vi "CAN Main.vi"(8 "error in (no error)":errorcluster, 10 "Interface":refnum<k21>="CAN1", 11 "Sequence Context In":refnum<k7>) -> (0 "error out":errorcluster)   [LabVIEW 2019, in "Wrappers.lvlib"]
uses:
  Wrappers.lvlib
  CAN/CAN.lvclass
  CAN/Setting.ctl
  <vilib>/addons/TestStand/_TSUtility.llb/TestStand - Set Property Value (Numeric Array).vi
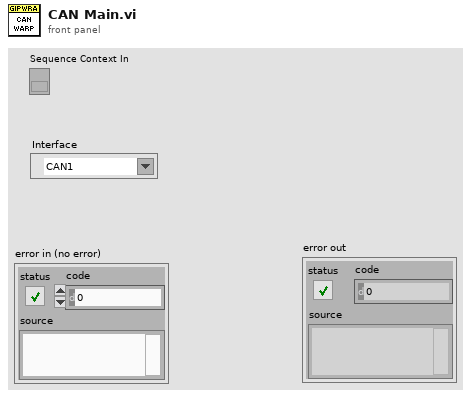
[diagram p1: front panel]
types:
  T1 = typedef "CAN.lvclass/Setting.ctl" = cluster{"Termination":u32, "Baud Rate":u64, "Interface":refnum<k21>, "XNET Database":refnum<k21>, "ECU":refnum<k21>}
  T2 = typedef "TestStand - Status Monitor.ctl" = cluster{"Sequence Context":refnum<k7>, "Execution":refnum<k7>, "Termination Monitor":refnum<k7>}
  T3 = cluster{"Send Tx":bool, "Stop":bool, "Rx Signals":string[], "Tx Signals":string[], "Tx Values In":dbl[]}
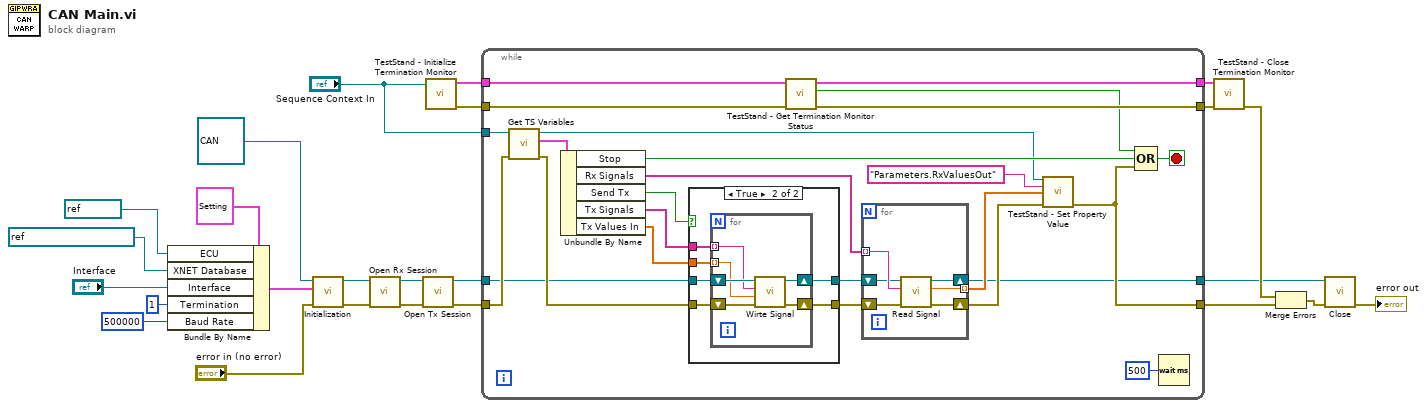
[diagram p0: block diagram]
diagram:
  n1 = Bundle By Name(cluster=T1 {"Termination"=1, "Baud Rate"=125000, "Interface"="CAN1", "XNET Database"="GIP_CAN_Database", "ECU"="GIP\nGIP_CAN_Database"} ("Setting"), "ECU"=refnum<k21> "GIP\ncan_messages_818", "XNET Database"=refnum<k21> "can_messages_818", "Interface"="Interface", "Termination"=u32 1, "Baud Rate"=u64 500000) -> (w11:T1)
  n2 = call "Initialization.vi"("error in (no error)"="error in (no error)", "Setting"=w11, "CAN in"=refnum<class "CAN.lvclass"> refnum ("CAN.lvclass")) -> ("error out"=w9:errorcluster, "CAN out"=w7:refnum<class "CAN.lvclass">)  [unwired: 7 in]
  n3 = call "Open Rx Session.vi"("error in (no error)"=w9, "CAN in"=w7) -> ("error out"=w8:errorcluster, "CAN out"=w6:refnum<class "CAN.lvclass">)  [unwired: 8 in]
  n4 = call "Open Tx Session.vi"("error in (no error)"=w8, "CAN in"=w6) -> ("error out"=w5:errorcluster, "CAN out"=w4:refnum<class "CAN.lvclass">)  [unwired: 8 in]
  n5 = call <vilib>:"TestStand - Initialize Termination Monitor.vi"("Sequence Context In"="Sequence Context In") -> ("error out"=w20:errorcluster, "Status Monitor Out"=w19:T2)  [unwired: 9 in]
  n6 = while {
    tunnel: w5 -> [w30]
    tunnel: w20 -> [w50]
    tunnel: w19 -> [w49]
    tunnel: [w48] -> w15
    tunnel: [w47] -> w18
    tunnel: "Sequence Context In" -> [w34]
    tunnel: [w42] -> w16
    tunnel: w4 -> [w29]
    tunnel: [w26] -> w1
    stop <- w46 stop-if-true
    n7 = call "Get TS Variables.vi"("error in (no error)"=w30, "Sequence Context In"=w34) -> ("error out"=w31:errorcluster, "Variables"=w32:T3, "Sequence Context Out"=w33:refnum<k7>)  [unwired: 7 in]
    n8 = Unbundle By Name(w32) -> ("Stop"=w43:bool, "Rx Signals"=w36:string[], "Send Tx"=w39:bool, "Tx Signals"=w40:string[], "Tx Values In"=w28:dbl[])
    n9 = case shown="True" w39 {
      tunnel: w31 -> [w52 w58]
      tunnel: [w52 w56] -> w38
      tunnel: w40 -> [_ w57]
      tunnel: w29 -> [w51 w55]
      tunnel: w28 -> [_ w54]
      tunnel: [w51 w53] -> w27
      frame False {
      }
      frame True {
        n10 = for {
          shift-right: [w63] -> w56
          shift-left: w58 -> [w64]
          tunnel: w57 -> [w61] mode=indexing
          tunnel: w54 -> [w60] mode=indexing
          shift-right: [w59] -> w53
          shift-left: w55 -> [w62]
          n11 = call "Wirte Signal.vi"("error in (no error)"=w64, "Signal Write"=w60, "Tx Signal In"=w61, "CAN in"=w62) -> ("error out"=w63:errorcluster, "CAN out"=w59:refnum<class "CAN.lvclass">)  [unwired: 6 in]
        }
      }
    }
    n12 = call <vilib>:"TestStand - Get Termination Monitor Status.vi"("error in (no error)"=w50, "Status Monitor In"=w49) -> ("error out"=w48:errorcluster, "Terminating or Aborting"=w45:bool, "Status Monitor Out"=w47:T2)  [unwired: 7 in]
    n13 = for {
      tunnel: w36 -> [w68] mode=indexing
      tunnel: [w66] -> w35 mode=indexing
      shift-right: [w69] -> w37
      shift-left: w38 -> [w70]
      shift-right: [w65] -> w26
      shift-left: w27 -> [w67]
      n14 = call "Read Signal.vi"("error in (no error)"=w70, "Rx Signal In"=w68, "CAN in"=w67) -> ("error out"=w69:errorcluster, "Signal out"=w66:dbl, "CAN out"=w65:refnum<class "CAN.lvclass">)  [unwired: 6 in]
    }
    n15 = call-poly <vilib>:"TestStand - Set Property Value.vi"("Sequence Context In"=w33, "Lookup String"="Parameters.RxValuesOut", "New Value"=w35, "error in (no error)"=w37) -> ("error out"=w42:errorcluster)  [unwired: 10 in, 1 out]
    n16 = Compound Arithmetic op=OR(w45, w43, w42) -> (w46:bool)
    n17 = Wait (ms)(milliseconds to wait=u32 500) -> ()  [unwired: 1 out]
  }
  n18 = call <vilib>:"TestStand - Close Termination Monitor.vi"("error in (no error)"=w15, "Status Monitor In"=w18) -> ("error out"=w14:errorcluster)  [unwired: 9 in]
  n19 = Merge Errors(w14, w16) -> (w3:errorcluster)
  n20 = call "Close.vi"("error in (no error)"=w3, "CAN in"=w1) -> ("error out"=→"error out":errorcluster)  [unwired: 8 in, 1 out]
